vi "Regenerate Hawkeye List.vi"() -> ()   [LabVIEW 2019, in "HawkeyeToolsMenu.lvlib"]
doc: "GUI to compare LabVIEW code between currently checked out branch with any other branch or any of its commits.\n\n(c) 2024 Soliton Technologies. All rights reserved."
uses:
  <vilib>/Hampel Software Engineering/Git API/Git API/GIT-api.lvclass
  <vilib>/Hampel Software Engineering/Git API/Git API/GIT-api.lvclass/GIT-api.ctl
  <vilib>/Hampel Software Engineering/Git API/Git API/Controls/GIT-Repository States.ctl
  <vilib>/Hampel Software Engineering/Git API/Git API/Accessors/GIT-Set Working Dir.vi
  <userlib>/_OpenG.lib/file/file.llb/File Exists - Scalar__ogtk.vi
  <userlib>/_OpenG.lib/file/file.llb/Valid Path - Traditional__ogtk.vi
  HawkeyeToolsMenu.lvlib
  vi.lib/Hawkeye/Hawkeye.lvlib
panel:
  in  "Tab Control":T1(tab)=enum."Main UI"
  out "Current Status":string
  in  "LVLib / LVClass / Sub Folder Path":path
  out "Status Indicator":string
  in  "Check Changed Libraries Only?":bool
  in  "Branch to Compare":string(combo)
  in  "Refresh Current Branch":bool
  out "Current Branch":string="origin/main"
  out "Current Branch Status":string
  in  "Stop":bool
  in  "Repo / Workspace Folder Path":path
  in  "Generate":bool
  # "1. Checkout the branch of interest in your system using any method - Git command line, Desktop Git GUI Clients etc.,\n\n2. Specify the local Repository Path.\n\n3. Verify the current branch, its status and select a branch or commit based on the Compare Mode and click on Compare to display the file changes.\n\n4. Double click on a file to initiate LabVIEW code comparison.\n\n5. Once done with required comparisons, exit the tool by closing the window. The tool cleans up the temporary files added during comparison.\n\n\nNote:\n1. This tool uses LabVIEW's VI Comparison Tool which requires LabVIEW Professional Development System.\n2. It is recommended to not use other Git Clients actively when comparing files using this tool to avoid Git command related errors.\n3. It is recommended to commit all changes (working copy) before using this tool for comparison."
  # "This tool uses git diff command to identify the changes. Hence it is recommended to commit all the changes (working copy) to have them considered for comparison. For code comparison, this tool uses LabVIEW's built in VI Comparison Tool.\n\nExample: Identify changes in current branch when comparing with other branch\n\n---A---B---C---D    <== other branch\n               \\\n                 E---F      <== current branch\n\n1. We will need to identify only the file changes introduced by current branch. E and F commits are those changes in the above example (commits after the common ancestor B).\n2. For the identified file changes compare with the other branch (D) to see how it differs. These differences will be our current branch changelist.\n\nWhy only current branch changes?\nIt is most useful to see how the current branch will modify the files when it is getting merged. Best use case for displaying only current branch changelist will be for Pull Request reviews."
  # "1. Repository Path - Local repository path (the top level folder with '.git' hidden folder in it). Git API will be initialized for this repository.\n\n2. Current Branch - Currently checked out branch. The status of the current branch is also displayed at top right. Click Refresh button to update the current branch if it is changed in the system or received new changes via Git Pull.\n\n3. Compare Mode - Select the type of comparison. You can compare the current branch with another branch or with a particular commit of a selected branch.\n\nIn branch comparison mode, you can enter the branch name for comparison in Branch to Compare. Remote branches usually start with \"origin/\" and local branches do not have \"origin/\" prefix. The branch's recent commit is displayed in Recent Commit and its details in Commit Details for reference. \n\nIn commit comparison mode, the commits available in the branch selected in Select Branch are listed in Commit to Compare. For the commit selected in Commit to Compare, its details will be displayed in the Commit Details. Use Commits to Fetch to limit the number of commits obtained and improve the loading time.\n\n     Note: Git doesn't maintain information on when the branch is created. So, all the commits of the selected branch will be displayed (all the way up to the very first commit after repository creation). Without a limit, it increases loading time.\n\n4. Compare - Identifies the file changes and Current Branch Changelist table shows the list of all files that are different in the current branch compared to the branch/commit selected.\n\n     Note: The other branch/commit in comparison would have introduced its own changes that are not part of current branch. Those changes will not be displayed.\n\n5. Filter LabVIEW VI and Control Files - Filter files except VI and CTL files. These require LabVIEW to compare but project, library and classes are text files that can be easily reviewed in the desktop Git GUI clients or in Pull Request of Git web services.\n\n6. LabVIEW Compare Options - Options to decide what to compare in the code. Set the required options before initiating code compare.\n\n7. Double click on the file you wish to compare. LabVIEW opens the compare window for the file from the current branch and the file from the other branch/commit (file will be suffixed with TEMP). It may take a while if the VI/CTL have lot of dependencies to load. Having the project pre-opened and opening this tool from that instance may reduce the loading time. Note that the file from the other branch/commit in comparison may be missing its dependent files which may not be available in the current branch or deleted in the current branch commits. This will cause the file to be in a broken state but does not affect the comparison. Another reason for the broken state may be due to the parent library/class not recognizing this new file with the suffix but this as well will not affect the comparison.\n\n     Note: The files from other branch/commit are placed at the same location in the current branch so that the LabVIEW can load the dependencies appropriately.\n\n8. Viewed Status (mixed checkbox) - A tick mark appears for every file compared or opened. Use the mixed checkbox (below the Current Branch Changelist) to control status for all files.\n\n     Note: Viewed status is only a visual aid for tracking and does not have any other function other than that.\n\n9. Panel Close - Stops the tools execution after removing all the new files introduced into the current branch (TEMP files)."
  # "This GUI allows you to regenerate dependency lists for the entire repository or for a selected folder, LabVIEW library (.lvlib), or LabVIEW class (.lvclass), ensuring dependency information is up to date."
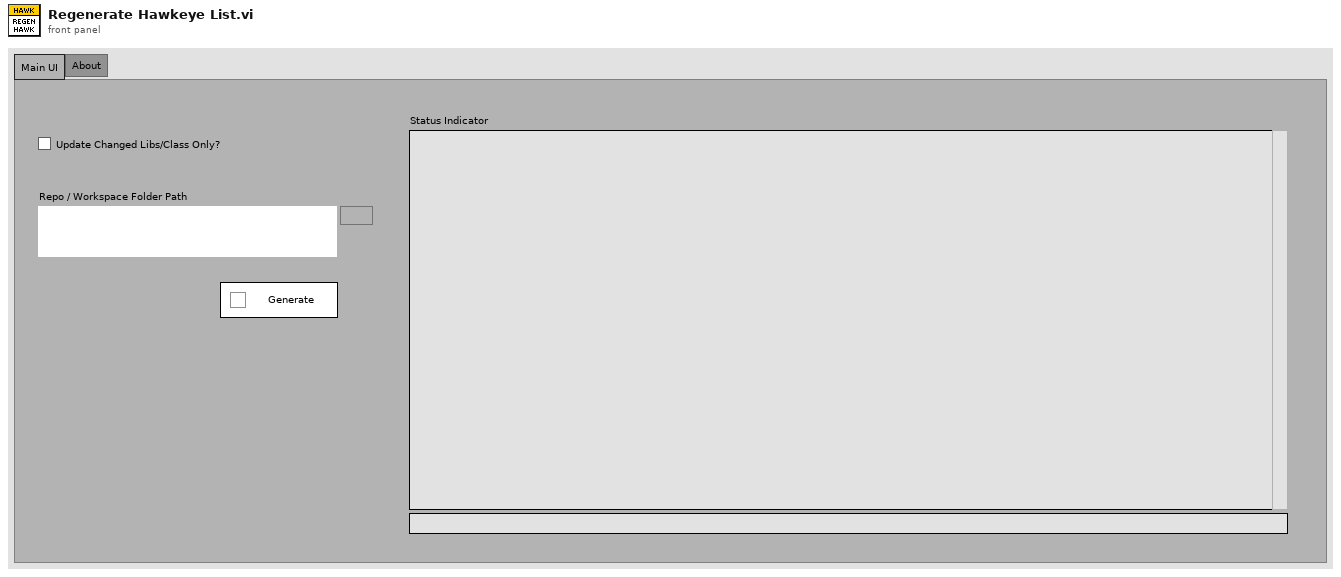
[diagram p1: front panel]
types:
  T1 = enum32{"Getting Started", "How it Works?", "Main UI", "Help", "About"}
  T2 = cluster{"Repository Path":path, "Git API Object":refnum<class "GIT-api.lvclass">, "Git API Initialized?":bool, "Current Branch":string, "Branch to Compare":string, "Check Changed Libraries Only?":bool, "Source Folder Path":path, "Build Specs Folder Path":path}
  T3 = typedef "GIT-API-for-LabVIEW.lvlib/GIT-api.lvclass/GIT-Repository States.ctl" = enum16{"up-to-date", "behind", "ahead", "diverged", "unpublished", "detached", "unknown"}
  T4 = enum8{"Enabled", "Disabled", "Disabled and Grayed Out"}
  T5 = typedef "Hawkeye.lvlib/HawkeyePathConfigs.ctl" = cluster{"GlobalIncludePaths":path[], "GlobalExcludePaths":path[], "BuildSpecsIncludePaths":path[], "ActualDepsIncludePaths":path[], "WorkspacePath":path, "SourceFolderPaths":path[], "ChangedFilesLogpaths":map{string, path}, "CacheRecreateDuration":dbl}
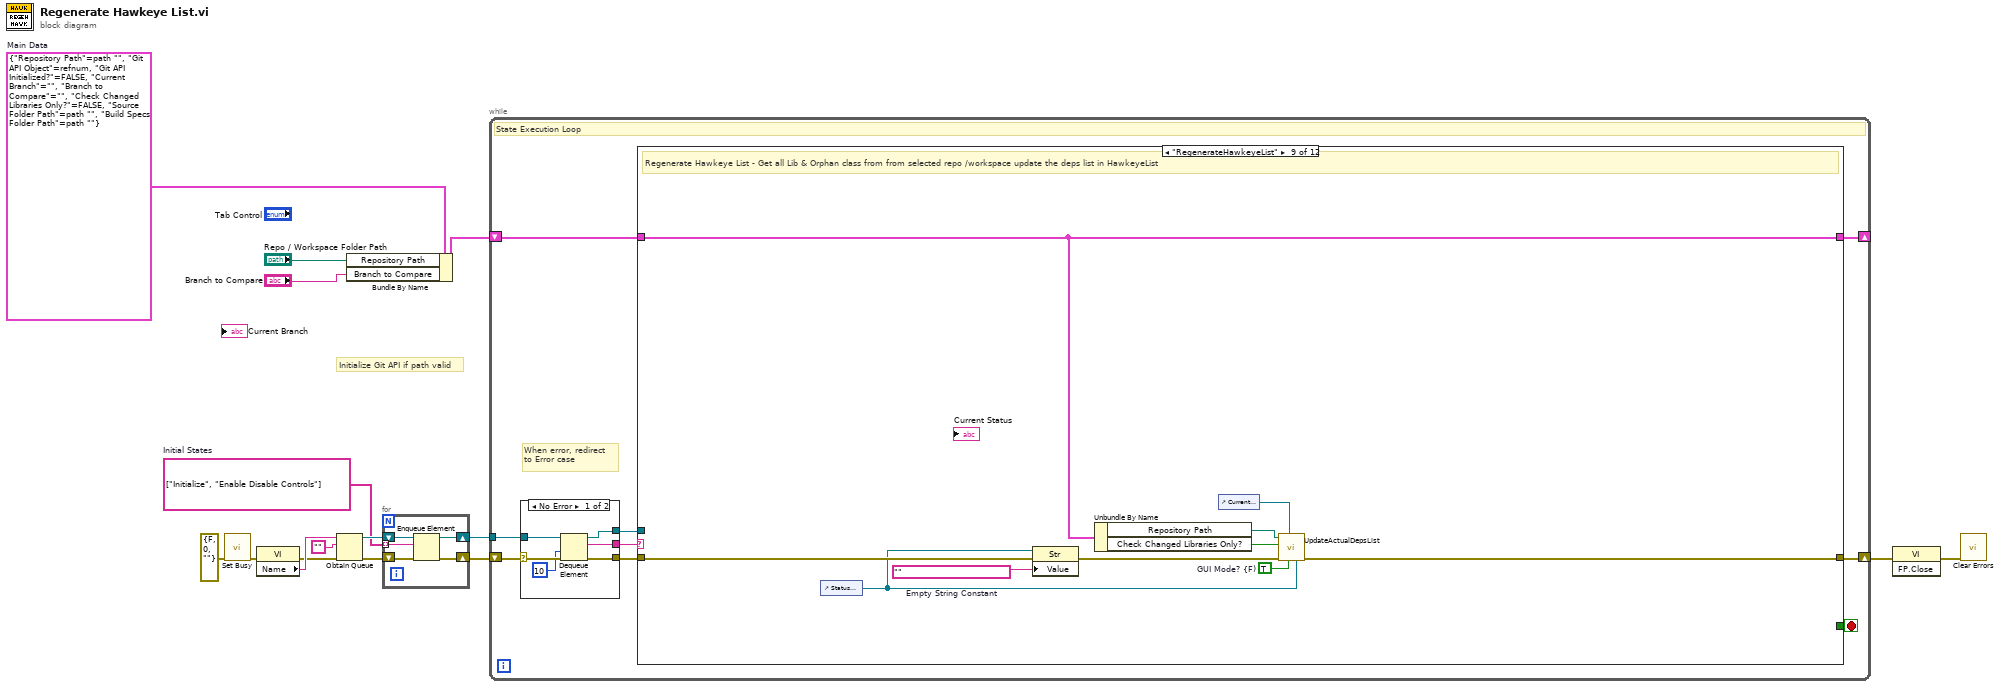
[diagram p0: block diagram]
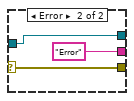
[diagram p2: hidden frame]
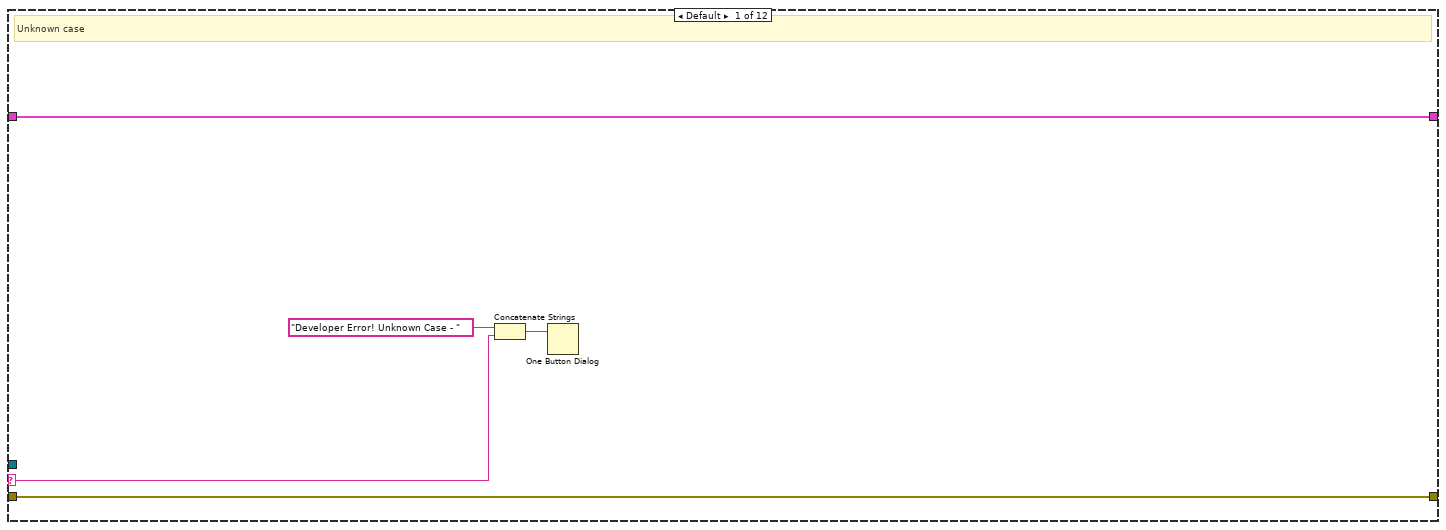
[diagram p3: hidden frame]
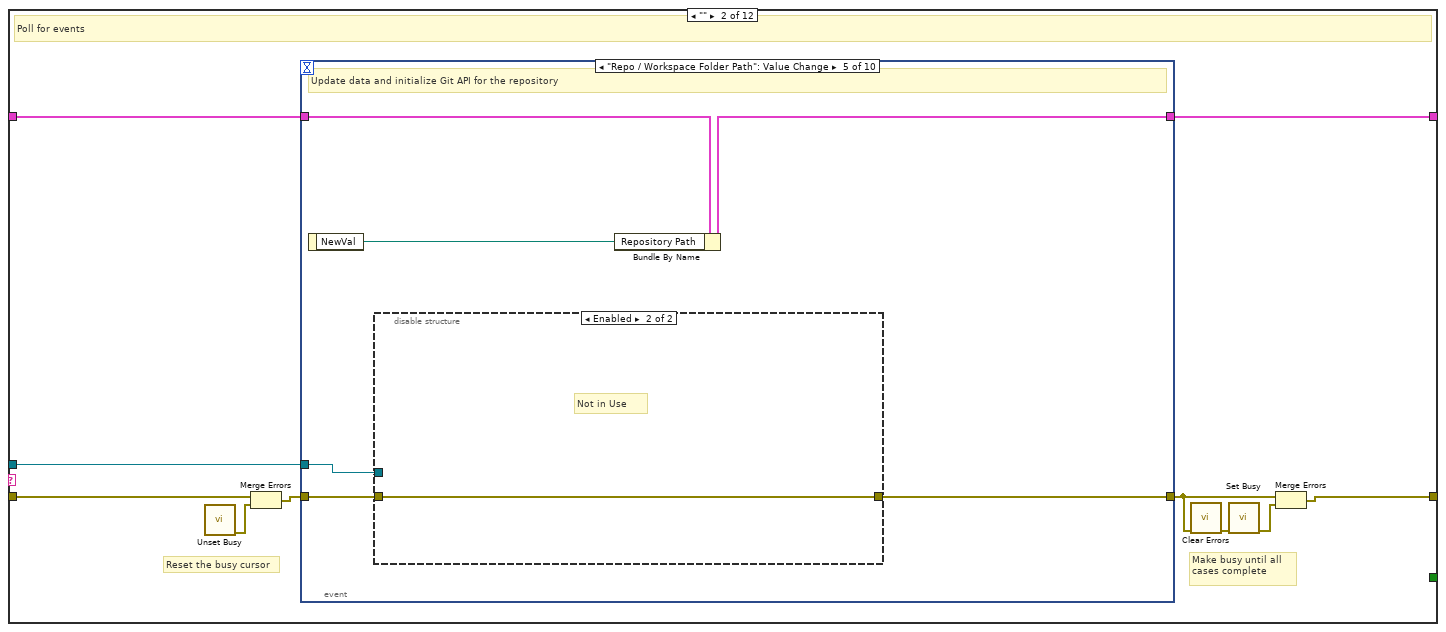
[diagram p4: hidden frame]
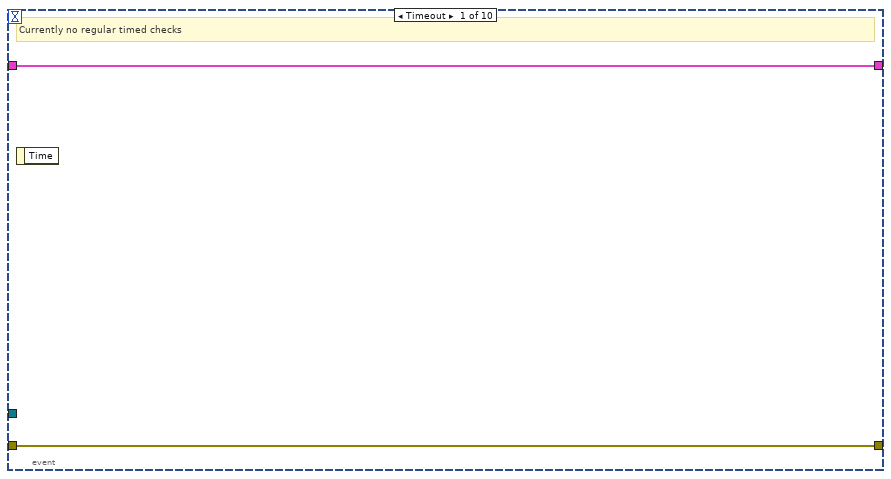
[diagram p5: hidden frame]
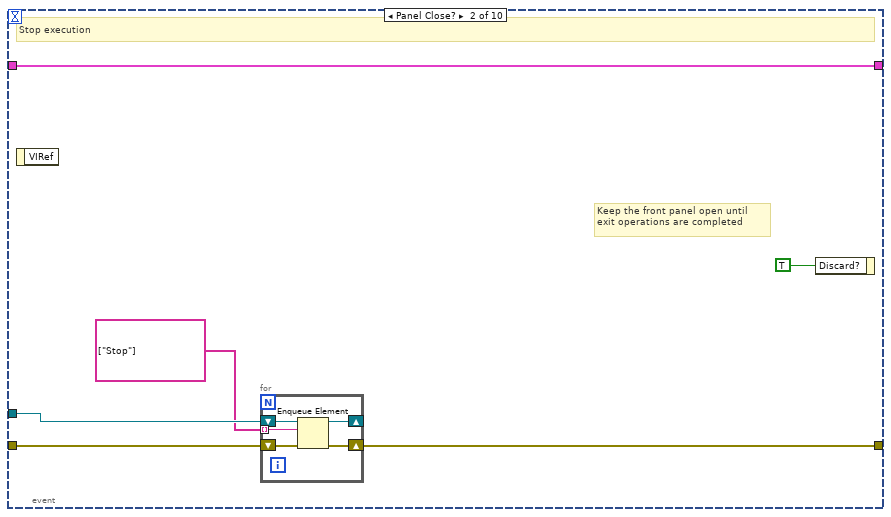
[diagram p6: hidden frame]
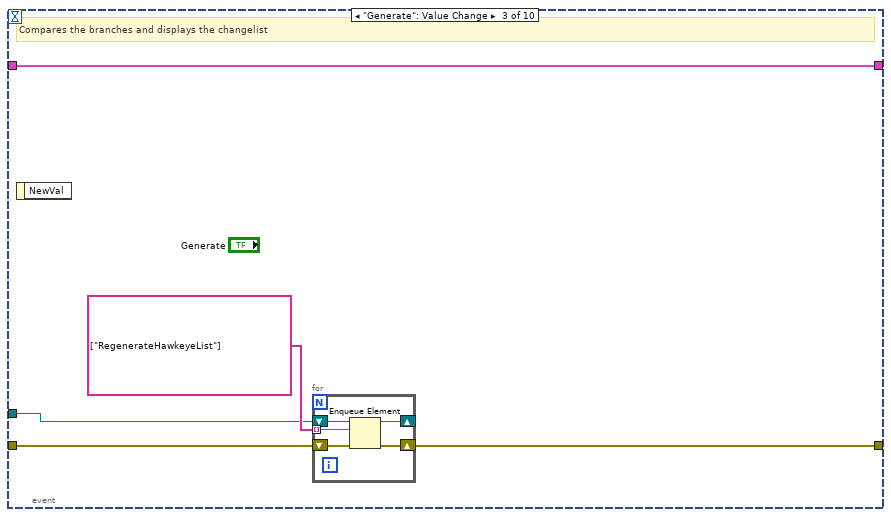
[diagram p7: hidden frame]
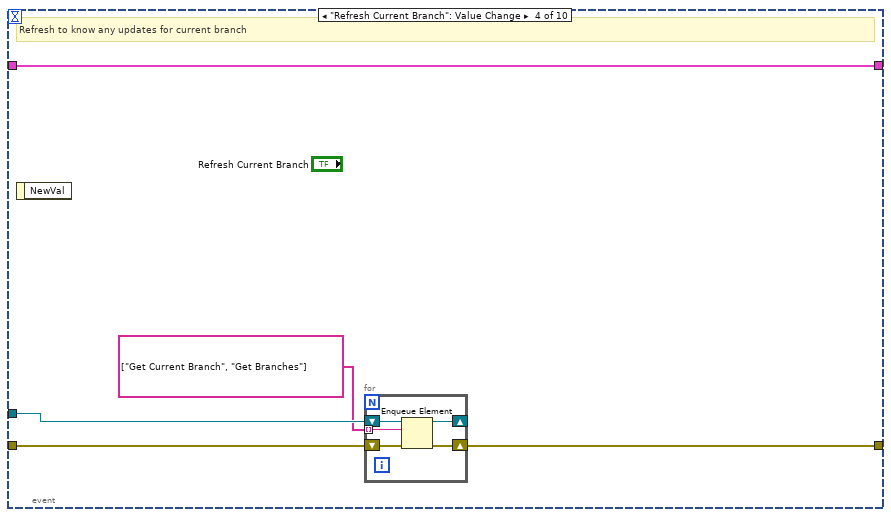
[diagram p8: hidden frame]
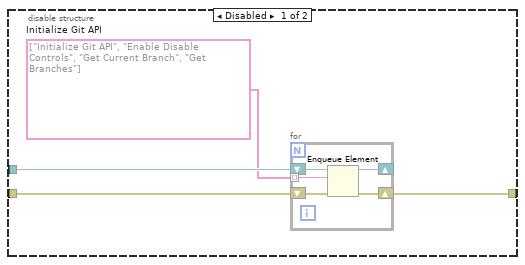
[diagram p9: hidden frame]
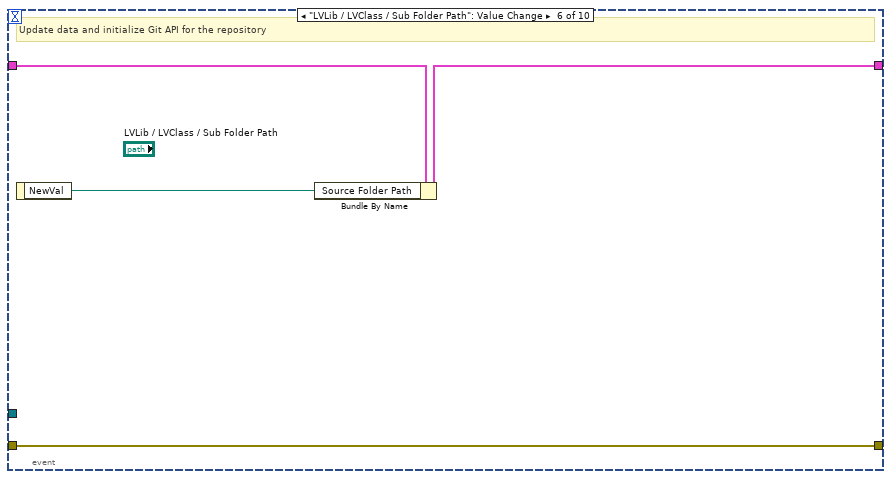
[diagram p10: hidden frame]
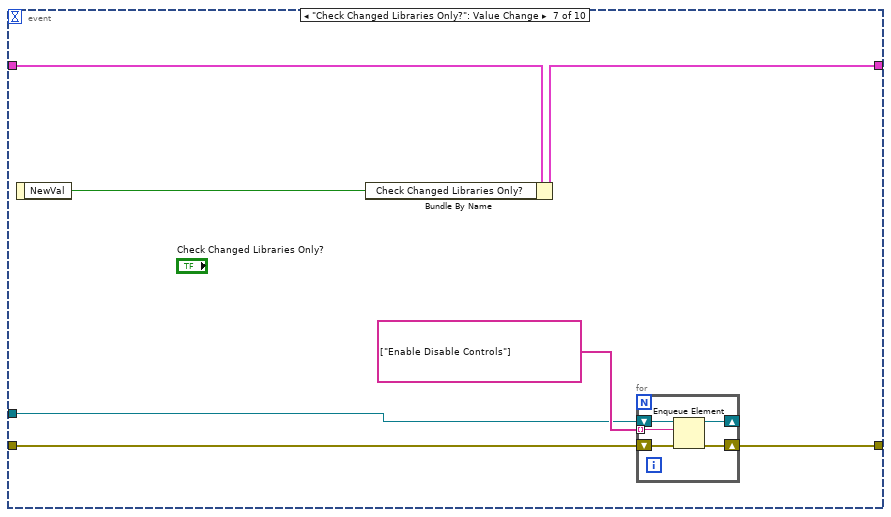
[diagram p11: hidden frame]
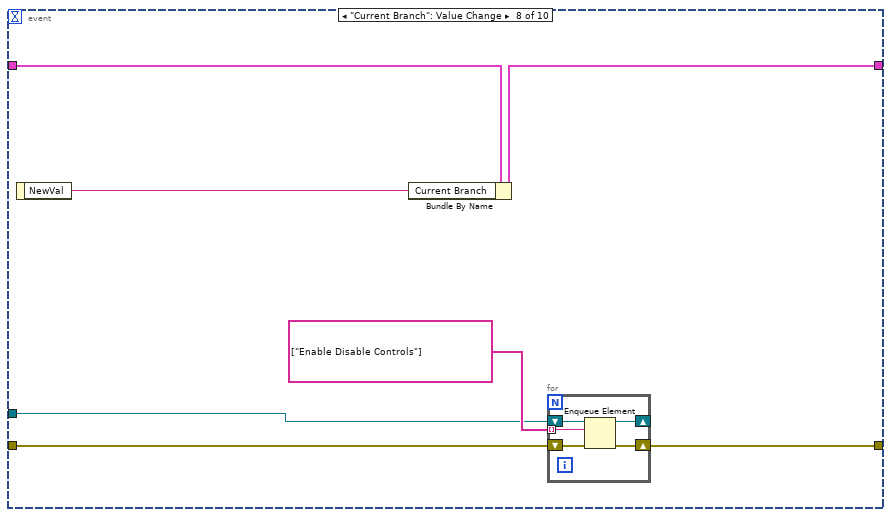
[diagram p12: hidden frame]
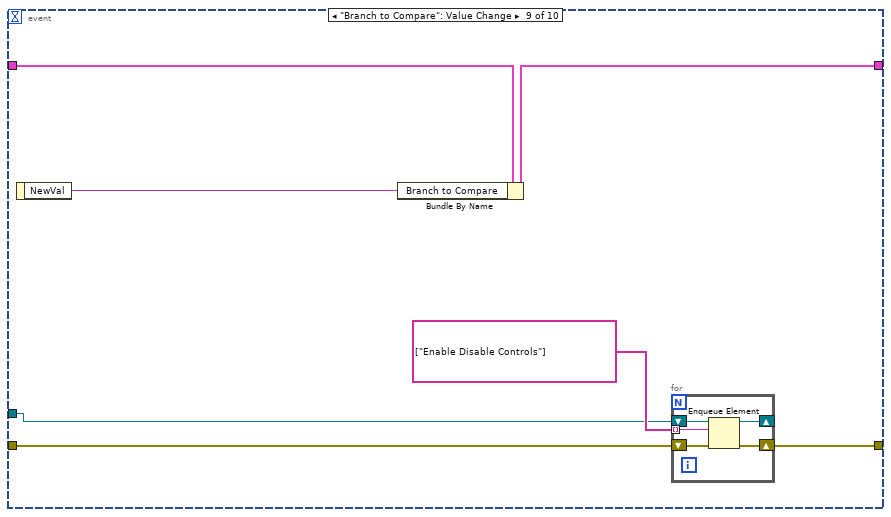
[diagram p13: hidden frame]
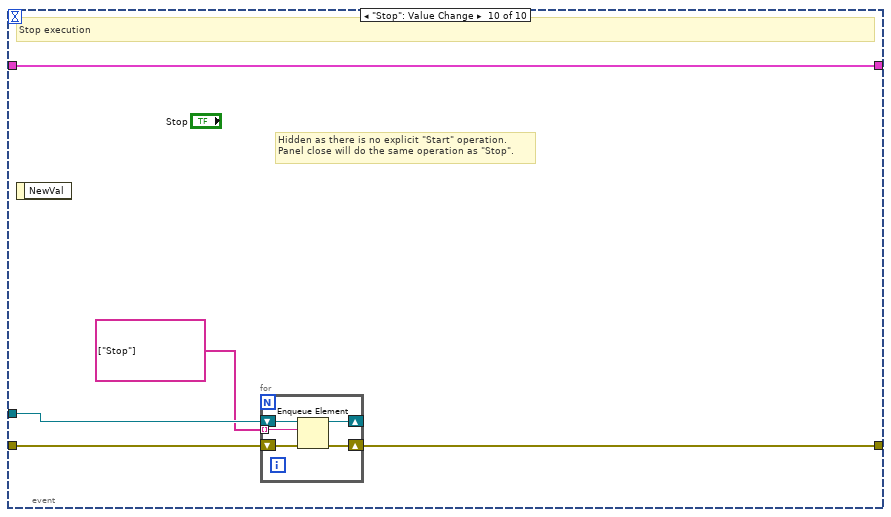
[diagram p14: hidden frame]
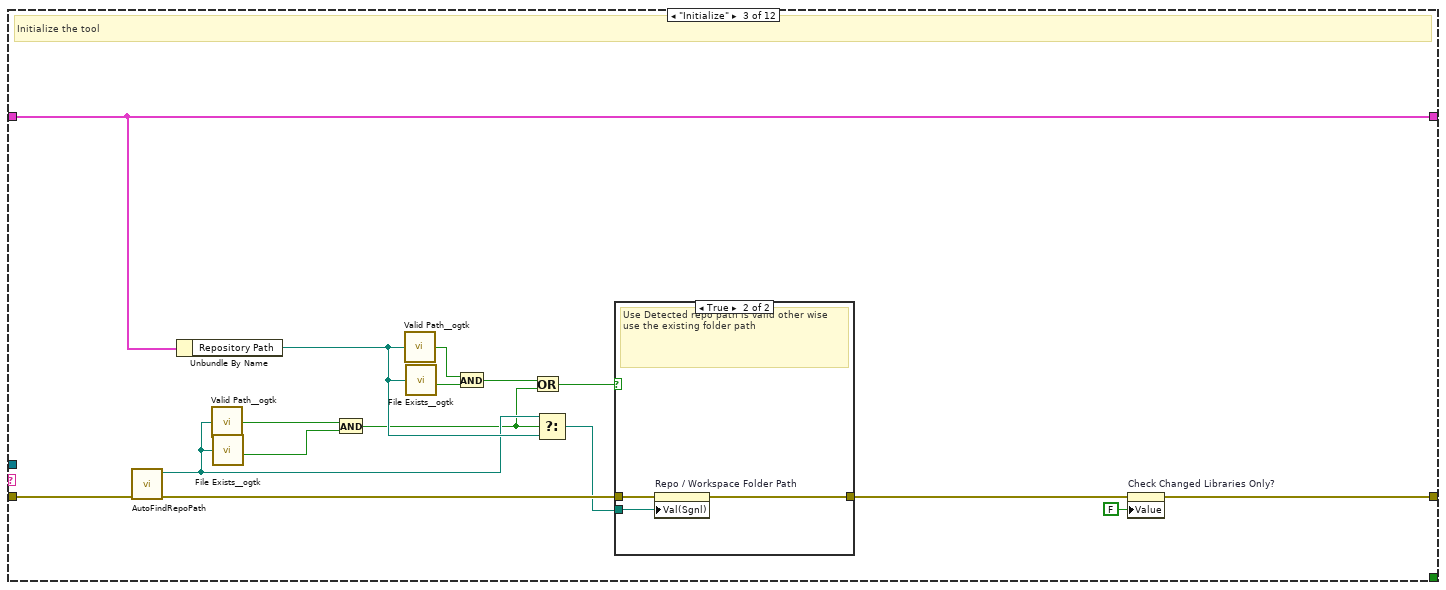
[diagram p15: hidden frame]
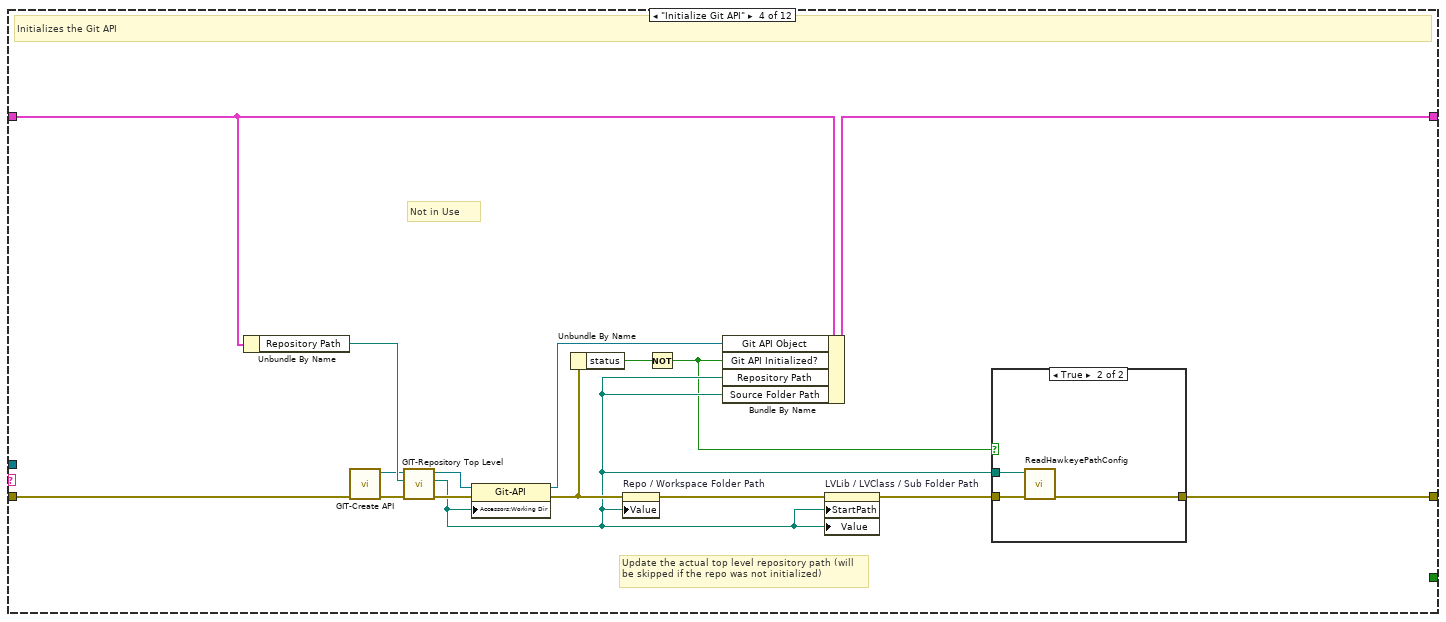
[diagram p17: hidden frame]
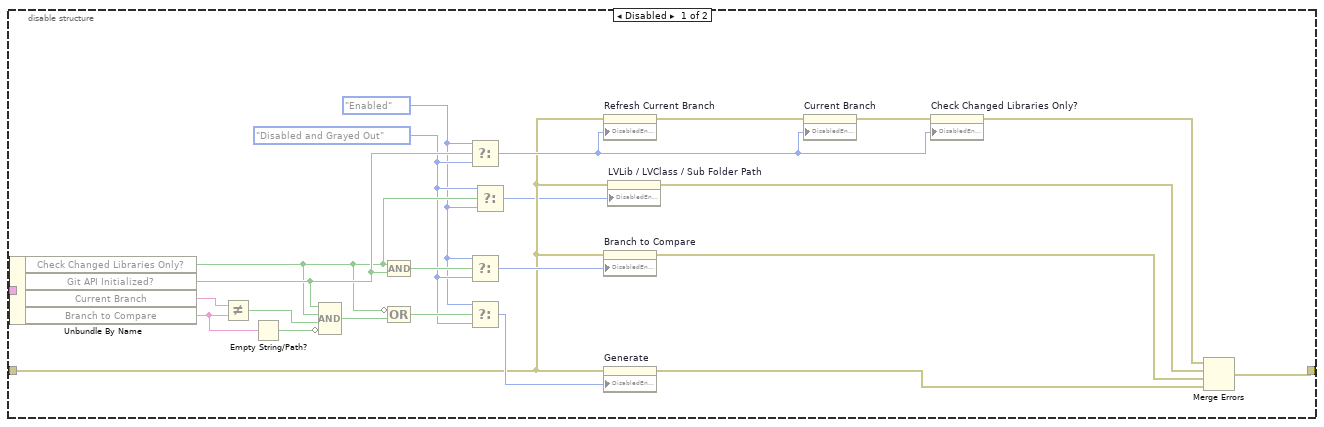
[diagram p20: hidden frame]
diagram:
  w1 = string[] ["Initialize", "Enable Disable Controls"]  # Initial States
  w13 = T2 {"Repository Path"=path "", "Git API Object"=refnum, "Git API Initialized?"=FALSE, "Current Branch"="", "Branch to Compare"="", "Check Changed Libraries Only?"=FALSE, "Source Folder Path"=path "", "Build Specs Folder Path"=path ""}  # Main Data
  # "Initialize Git API if path valid"
  n1 = call <vilib>:"Set Busy.vi"("error in (no error)"=errorcluster {"status"=FALSE, "code"=0, "source"=""}) -> ("error out"=w6:errorcluster)  [unwired: 9 in, 1 out]
  n2 = property class="VI"(error in=w6) -> (error out=w15:errorcluster, "Name"=w16:string)  [unwired: 1 in, 1 out]
  n3 = Obtain Queue(name (unnamed)=w16, element data type="", error in (no error)=w15) -> (queue out=w11:refnum<queue>, error out=w8:errorcluster)  [unwired: 2 in, 1 out]
  n4 = Bundle By Name(cluster=w13, "Repository Path"="Repo / Workspace Folder Path", "Branch to Compare"="Branch to Compare") -> (w12:T2)
  n5 = for {
    tunnel: w1 -> [w18] mode=indexing
    shift-right: [w20] -> w10
    shift-left: w8 -> [w21]
    shift-right: [w17] -> w9
    shift-left: w11 -> [w19]
    n6 = Enqueue Element(queue=w19, element=w18, error in (no error)=w21) -> (queue out=w17:refnum<queue>, error out=w20:errorcluster)  [unwired: 1 in, 1 out]
  }
  n7 = while {
    shift-right: [w22] -> w4
    shift-left: w10 -> [w24]
    tunnel: w9 -> [w25]
    shift-right: [w27] -> _
    shift-left: w12 -> [w26]
    stop <- w28 stop-if-true
    # "When error, redirect to Error case"
    # "State Execution Loop"
    n8 = case shown="No Error" w24 {
      selector: w24 -> [w33 w37]
      tunnel: [w36 "Error" ("element")] -> w30
      tunnel: [w35 w39] -> w29
      tunnel: w25 -> [w34 w39]
      tunnel: [w31 w37] -> w23
      frame No Error {
        n9 = Dequeue Element(queue=w34, timeout in ms (-1)=10, error in (no error)=w33) -> (queue out=w35:refnum<queue>, element=w36:string, error out=w31:errorcluster)  [unwired: 1 out]
      }
      frame Error {
      }
    }
    n10 = case shown="\"RegenerateHawkeyeList\"" w30 {
      selector: w30 -> [w43 _ _ _ _ _ _ _ _ _ _ _]
      tunnel: w23 -> [w41 w48 w166 w189 w194 w227 w273 w303 w324 w333 w343 w351]
      tunnel: w29 -> [_ w54 _ _ _ _ _ _ _ w331 w340 w348]
      tunnel: [w41 w50 w169 w175 w195 w236 w282 w299 w325 w332 w339 w344] -> w22
      tunnel: [_ _ _ _ _ _ _ _ _ _ w341 _] -> w28
      tunnel: [w40 w52 w163 w186 w196 w239 w280 w304 w328 w330 w342 w352] -> w27
      tunnel: w26 -> [w40 w53 w163 w188 w196 w240 w281 w304 w328 w330 w342 w352]
      frame Default {
        # "Unknown case"
        n11 = Concatenate Strings("Developer Error! Unknown Case - " ("string"), w43) -> (w42:string)
        n12 = One Button Dialog(message=w42) -> ()  [unwired: 1 in, 1 out]
      }
      frame "" {
        # "Reset the busy cursor"
        # "Make busy until all cases complete"
        # "Poll for events"
        n13 = call <vilib>:"Unset Busy.vi"() -> ("error out"=w49:errorcluster)  [unwired: 11 in]
        n14 = Merge Errors(w48, w49) -> (w47:errorcluster)
        n15 = event shown="[4] \"Repo / Workspace Folder Path\": Value Change" {
          selector: _ -> [_ _ _ _ _ _ _ _ _ _]
          dyn-events: _ -> [_ _ _ _ _ _ _ _ _ _]
          timeout: _ -> [_ _ _ _ _ _ _ _ _ _]
          tunnel: w47 -> [w55 w62 w71 w82 w90 w104 w109 w120 w132 w148]
          tunnel: w54 -> [_ w61 w70 w81 w89 _ w108 w122 w134 w147]
          tunnel: [w55 w60 w69 w79 w88 w104 w110 w121 w133 w146] -> w46
          tunnel: w53 -> [w56 w59 w68 w78 w93 w107 w114 w126 w138 w145]
          tunnel: [w56 w59 w68 w78 w92 w106 w113 w125 w137 w145] -> w52
          event Timeout {
            # "Currently no regular timed checks"
            n16 = event-data() -> ()  [unwired: 1 in, 1 out]
          }
          event Panel Close? {
            # "Keep the front panel open until exit operations are completed"
            # "Stop execution"
            n17 = event-data() -> ()  [unwired: 1 in, 1 out]
            n18 = for {
              tunnel: string[] ["Stop"] -> [w64] mode=indexing
              shift-right: [w66] -> w60
              shift-left: w62 -> [w67]
              shift-right: [w63] -> _
              shift-left: w61 -> [w65]
              n19 = Enqueue Element(queue=w65, element=w64, error in (no error)=w67) -> (queue out=w63:refnum<queue>, error out=w66:errorcluster)  [unwired: 1 in, 1 out]
            }
            n20 = event-data("Discard?"=TRUE) -> ()  [unwired: 1 in, 1 out]
          }
          event "Generate": Value Change {
            # "Compares the branches and displays the changelist"
            n21 = event-data() -> ()  [unwired: 1 in, 1 out]
            n22 = for {
              tunnel: string[] ["RegenerateHawkeyeList"] -> [w74] mode=indexing
              shift-right: [w76] -> w69
              shift-left: w71 -> [w77]
              shift-right: [w73] -> _
              shift-left: w70 -> [w75]
              n23 = Enqueue Element(queue=w75, element=w74, error in (no error)=w77) -> (queue out=w73:refnum<queue>, error out=w76:errorcluster)  [unwired: 1 in, 1 out]
            }
          }
          event "Refresh Current Branch": Value Change {
            # "Refresh to know any updates for current branch"
            n24 = event-data() -> ()  [unwired: 1 in, 1 out]
            n25 = for {
              tunnel: string[] ["Get Current Branch", "Get Branches"] -> [w84] mode=indexing
              shift-right: [w86] -> w79
              shift-left: w82 -> [w87]
              shift-right: [w83] -> _
              shift-left: w81 -> [w85]
              n26 = Enqueue Element(queue=w85, element=w84, error in (no error)=w87) -> (queue out=w83:refnum<queue>, error out=w86:errorcluster)  [unwired: 1 in, 1 out]
            }
          }
          event "Repo / Workspace Folder Path": Value Change {
            # "Update data and initialize Git API for the repository"
            n27 = event-data() -> ("NewVal"=w91:path)  [unwired: 1 in]
            n28 = disable-structure shown="Enabled" {
              disable-tunnel: w90 -> [w97 w103]
              disable-tunnel: w89 -> [w96 _]
              disable-tunnel: [w95 w103] -> w88
              frame Disabled {
                w94 = string[] ["Initialize Git API", "Enable Disable Controls", "Get Current Branch", "Get Branches"]  # Initialize Git API
                n29 = for {
                  tunnel: w94 -> [w99] mode=indexing
                  shift-right: [w101] -> w95
                  shift-left: w97 -> [w102]
                  shift-right: [w98] -> _
                  shift-left: w96 -> [w100]
                  n30 = Enqueue Element(queue=w100, element=w99, error in (no error)=w102) -> (queue out=w98:refnum<queue>, error out=w101:errorcluster)  [unwired: 1 in, 1 out]
                }
              }
              frame Enabled {
                # "Not in Use"
              }
            }
            n31 = Bundle By Name(cluster=w93, "Repository Path"=w91) -> (w92:T2)
          }
          event "LVLib / LVClass / Sub Folder Path": Value Change {
            # "Update data and initialize Git API for the repository"
            n32 = event-data() -> ("NewVal"=w105:path)  [unwired: 1 in]
            n33 = Bundle By Name(cluster=w107, "Source Folder Path"=w105) -> (w106:T2)
          }
          event "Check Changed Libraries Only?": Value Change {
            n34 = event-data() -> ("NewVal"=w112:bool)  [unwired: 1 in]
            n35 = Bundle By Name(cluster=w114, "Check Changed Libraries Only?"=w112) -> (w113:T2)
            n36 = for {
              tunnel: string[] ["Enable Disable Controls"] -> [w116] mode=indexing
              shift-right: [w118] -> w110
              shift-left: w109 -> [w119]
              shift-right: [w115] -> _
              shift-left: w108 -> [w117]
              n37 = Enqueue Element(queue=w117, element=w116, error in (no error)=w119) -> (queue out=w115:refnum<queue>, error out=w118:errorcluster)  [unwired: 1 in, 1 out]
            }
          }
          event "Current Branch": Value Change {
            n38 = event-data() -> ("NewVal"=w124:string)  [unwired: 1 in]
            n39 = Bundle By Name(cluster=w126, "Current Branch"=w124) -> (w125:T2)
            n40 = for {
              tunnel: string[] ["Enable Disable Controls"] -> [w128] mode=indexing
              shift-right: [w130] -> w121
              shift-left: w120 -> [w131]
              shift-right: [w127] -> _
              shift-left: w122 -> [w129]
              n41 = Enqueue Element(queue=w129, element=w128, error in (no error)=w131) -> (queue out=w127:refnum<queue>, error out=w130:errorcluster)  [unwired: 1 in, 1 out]
            }
          }
          event "Branch to Compare": Value Change {
            n42 = event-data() -> ("NewVal"=w136:string)  [unwired: 1 in]
            n43 = Bundle By Name(cluster=w138, "Branch to Compare"=w136) -> (w137:T2)
            n44 = for {
              tunnel: string[] ["Enable Disable Controls"] -> [w140] mode=indexing
              shift-right: [w142] -> w133
              shift-left: w132 -> [w143]
              shift-right: [w139] -> _
              shift-left: w134 -> [w141]
              n45 = Enqueue Element(queue=w141, element=w140, error in (no error)=w143) -> (queue out=w139:refnum<queue>, error out=w142:errorcluster)  [unwired: 1 in, 1 out]
            }
          }
          event "Stop": Value Change {
            # "Hidden as there is no explicit \"Start\" operation.\nPanel close will do the same operation as \"Stop\"."
            # "Stop execution"
            n46 = event-data() -> ()  [unwired: 1 in, 1 out]
            n47 = for {
              tunnel: string[] ["Stop"] -> [w150] mode=indexing
              shift-right: [w152] -> w146
              shift-left: w148 -> [w153]
              shift-right: [w149] -> _
              shift-left: w147 -> [w151]
              n48 = Enqueue Element(queue=w151, element=w150, error in (no error)=w153) -> (queue out=w149:refnum<queue>, error out=w152:errorcluster)  [unwired: 1 in, 1 out]
            }
          }
        }
        n49 = call <vilib>:"Clear Errors.vi"("error in (no error)"=w46) -> ("error out"=w45:errorcluster)  [unwired: 5 in, 1 out]
        n50 = call <vilib>:"Set Busy.vi"("error in (no error)"=w45) -> ("error out"=w51:errorcluster)  [unwired: 9 in, 1 out]
        n51 = Merge Errors(w46, w51) -> (w50:errorcluster)
      }
      frame "Initialize" {
        # "Initialize the tool"
        n52 = call "AutoFindRepoPath.vi"("error in (no error)"=w166) -> ("error out"=w167:errorcluster, "Repo Path"=w157:path)  [unwired: 9 in]
        n53 = Unbundle By Name(w163) -> ("Repository Path"=w159:path)
        n54 = call-poly <userlib>:"Valid Path__ogtk.vi"("path"=w157) -> ("valid"=w164:bool)
        n55 = call-poly <userlib>:"File Exists__ogtk.vi"("file path"=w157) -> ("exists"=w165:bool)  [unwired: 6 in, 1 out]
        n56 = And(x=w164, y=w165) -> (x .and. y?=w156:bool)
        n57 = call-poly <userlib>:"Valid Path__ogtk.vi"("path"=w159) -> ("valid"=w158:bool)
        n58 = call-poly <userlib>:"File Exists__ogtk.vi"("file path"=w159) -> ("exists"=w162:bool)  [unwired: 6 in, 1 out]
        n59 = And(x=w158, y=w162) -> (x .and. y?=w161:bool)
        n60 = Or(x=w161, y=w156) -> (x .or. y?=w160:bool)
        n61 = Select(t=w157, s=w156, f=w159) -> (s? t:f=w154:path)
        n62 = case shown="True" w160 {
          tunnel: w167 -> [w170 w173]
          tunnel: [w170 w171] -> w155
          tunnel: w154 -> [_ w172]
          frame False {
          }
          frame True {
            # "Use Detected repo path is valid other wise use the existing folder path"
            n63 = property on="Repo / Workspace Folder Path" class="Path"(error in=w173, "Val(Sgnl)"=w172) -> (error out=w171:errorcluster)  [unwired: 1 in, 1 out]
          }
        }
        n64 = property on="Check Changed Libraries Only?" class="Bool (strict)"(error in=w155, "Value"=FALSE ("Check Changed Libraries Only?")) -> (error out=w169:errorcluster)  [unwired: 1 in, 1 out]
      }
      frame "Initialize Git API" {
        # "Not in Use"
        # "Update the actual top level repository path (will be skipped if the repo was not initialized)"
        # "Initializes the Git API"
        n65 = Unbundle By Name(w188) -> ("Repository Path"=w185:path)
        n66 = call <vilib>:"GIT-Create API.vi"("error in"=w189) -> ("error out"=w184:errorcluster, "git-api out"=w182:refnum<class "GIT-api.lvclass">)  [unwired: 9 in]
        n67 = call <vilib>:"GIT-Repository Top Level.vi"("error in"=w184, "Current Path"=w185, "git-api in"=w182) -> ("error out"=w181:errorcluster, "Repo Top Level Path"=w177:path, "git-api out"=w183:refnum<class "GIT-api.lvclass">)  [unwired: 6 in]
        n68 = property class="Git-API"(reference=w183, error in=w181, "Accessors:Working Dir"=w177) -> (reference out=w187:refnum<class "GIT-api.lvclass">, error out=w179:errorcluster)
        n69 = Unbundle By Name(w179) -> ("status"=w180:bool)
        n70 = property on="Repo / Workspace Folder Path" class="Path"(error in=w179, "Value"=w177) -> (error out=w178:errorcluster)  [unwired: 1 in, 1 out]
        n71 = Not(x=w180) -> (.not. x?=w174:bool)
        n72 = Bundle By Name(cluster=w188, "Git API Object"=w187, "Git API Initialized?"=w174, "Repository Path"=w177, "Source Folder Path"=w177) -> (w186:T2)
        n73 = property on="LVLib / LVClass / Sub Folder Path" class="Path"(error in=w178, "StartPath"=w177, "Value"=w177) -> (error out=w176:errorcluster)  [unwired: 1 in, 1 out]
        n74 = case shown="True" w174 {
          tunnel: w177 -> [_ w193]
          tunnel: w176 -> [w190 w192]
          tunnel: [w190 w191] -> w175
          frame False {
          }
          frame True {
            n75 = call "ReadHawkeyePathConfig.vi"("error in (no error)"=w192, "Workspace Path"=w193) -> ("error out"=w191:errorcluster)  [unwired: 8 in, 1 out]
          }
        }
      }
      frame "Enable Disable Controls" {
        # "Enable or disable controls based on Git API initialized or not"
        n76 = disable-structure shown="Enabled" {
          disable-tunnel: w196 -> [w220 _]
          disable-tunnel: [w219 w221] -> w195
          disable-tunnel: w194 -> [w202 w221]
          frame Disabled {
            w199 = T4."Disabled and Grayed Out" ("Disabled")
            w198 = T4."Enabled" ("Disabled")
            n77 = Unbundle By Name(w220) -> ("Check Changed Libraries Only?"=w200:bool, "Git API Initialized?"=w207:bool, "Current Branch"=w215:string, "Branch to Compare"=w211:string)
            n78 = Not Equal?(x=w215, y=w211) -> (x != y?=w208:bool)
            n79 = Empty String/Path?(string/path=w211) -> (empty?=w210:bool)
            n80 = Compound Arithmetic op=AND(w207, w200, w208, invert w210) -> (w209:bool)
            n81 = Compound Arithmetic op=AND(w200, w207) -> (w214:bool)
            n82 = Compound Arithmetic op=OR(invert w200, w209) -> (w216:bool)
            n83 = Select(t=w198, s=w207, f=w199) -> (s? t:f=w203:T4)
            n84 = Select(t=w198, s=w214, f=w199) -> (s? t:f=w213:T4)
            n85 = Select(t=w198, s=w216, f=w199) -> (s? t:f=w217:T4)
            n86 = Select(t=w199, s=w200, f=w198) -> (s? t:f=w197:T4)
            n87 = property on="Refresh Current Branch" class="Bool"(error in=w202, "DisabledEnum"=w203) -> (error out=w206:errorcluster)  [unwired: 1 in, 1 out]
            n88 = property on="Branch to Compare" class="CmbBox"(error in=w202, "DisabledEnum"=w213) -> (error out=w218:errorcluster)  [unwired: 1 in, 1 out]
            n89 = property on="Generate" class="Bool"(error in=w202, "DisabledEnum"=w217) -> (error out=w212:errorcluster)  [unwired: 1 in, 1 out]
            n90 = property on="LVLib / LVClass / Sub Folder Path" class="Path"(error in=w202, "DisabledEnum"=w197) -> (error out=w201:errorcluster)  [unwired: 1 in, 1 out]
            n91 = property on="Current Branch" class="Str"(error in=w206, "DisabledEnum"=w203) -> (error out=w205:errorcluster)  [unwired: 1 in, 1 out]
            n92 = property on="Check Changed Libraries Only?" class="Bool (strict)"(error in=w205, "DisabledEnum"=w203) -> (error out=w204:errorcluster)  [unwired: 1 in, 1 out]
            n93 = Merge Errors(w204, w201, w218, w212) -> (w219:errorcluster)
          }
          frame Enabled {
            # "Not in Use"
          }
        }
      }
      frame "Get Current Branch" {
        # "Not in Use"
        # "Fetch updates from all remotes"
        # "Identify the currently checked out branch and its status and update the UI control"
        n94 = Unbundle By Name(w240) -> ("Git API Object"=w228:refnum<class "GIT-api.lvclass">)
        n95 = call <vilib>:"GIT-Fetch.vi"("param"="--all", "error in"=w227, "git-api in"=w228) -> ("error out"=w233:errorcluster, "git-api out"=w234:refnum<class "GIT-api.lvclass">)  [unwired: 6 in, 1 out]
        n96 = call <vilib>:"GIT-Repository Status.vi"("error in"=w233, "git-api in"=w234) -> ("error out"=w242:errorcluster, "State"=w225:T3, "git-api out"=w241:refnum<class "GIT-api.lvclass">)  [unwired: 6 in, 1 out]
        n97 = call <vilib>:"GIT-Current Branch.vi"("error in"=w242, "git-api in"=w241) -> ("error out"=w226:errorcluster, "current branch"=w229:string)  [unwired: 7 in, 1 out]
        n98 = Equal?(x=GIT-Repository_States."detached", y=w225) -> (x = y?=w230:bool)
        n99 = Select(t="HEAD", s=w230, f=w229) -> (s? t:f=w222:string)
        n100 = Format Into String(format string="%s", error in=w226, w225) -> (resulting string=→"Current Branch Status":string, error out=w223:errorcluster)  [unwired: 1 in]
        n101 = case "Color for quick identification" shown="\"up-to-date\"" w225 {
          tunnel: [u32 32768 u32 16711680 u32 16860 u32 16744448 u32 16777222 u32 7171459 u32 16711680] -> w235
          frame "up-to-date" {
          }
          frame "behind" {
          }
          frame "ahead" {
          }
          frame "diverged" {
          }
          frame "unpublished" {
          }
          frame "detached" {
          }
          frame "unknown" {
          }
        }
        n102 = Bundle By Name(cluster=w240, "Current Branch"=w222) -> (w239:T2)
        n103 = property on="Current Branch Status" class="Str"(error in=w223, "Text.TextColor"=w235) -> (error out=w236:errorcluster)  [unwired: 1 in, 1 out]
      }
      frame "Get Branches" {
        w263 = 0  # Branch Name List
        w268 = string[][] []
        w267 = "%s" ("format string")
        # "Not in Use"
        # "Reset if previous value not found"
        # "Combine local and remote branches"
        # "List Local branches"
        # "List Remote branches\nNote: All remote branches usually start with origin/ unless renamed"
        # "Reset if previous value not found"
        # "Get all local and remote branches and update UI control"
        n104 = Unbundle By Name(w281) -> ("Current Branch"=w253:string, "Git API Object"=w271:refnum<class "GIT-api.lvclass">)
        n105 = call <vilib>:"GIT-Branch.vi"("error in"=w273, "git-api in"=w271) -> ("error out"=w272:errorcluster, "std out"=w264:string, "git-api out"=w265:refnum<class "GIT-api.lvclass">)  [unwired: 7 in]
        n106 = call <vilib>:"GIT-Branch.vi"("param"="-r", "error in"=w272, "git-api in"=w265) -> ("error out"=w275:errorcluster, "std out"=w266:string)  [unwired: 6 in, 1 out]
        n107 = Spreadsheet String To Array(format string=w267, spreadsheet string=w264, array type (2D Dbl)=w268) -> (array=w283:string[][])  [unwired: 1 in]
        n108 = Spreadsheet String To Array(format string=w267, spreadsheet string=w266, array type (2D Dbl)=w268) -> (array=w269:string[][])  [unwired: 1 in]
        n109 = Index Array(array=w283, index (col)=w263) -> (element=w270:string[])  [unwired: 1 in]
        n110 = Index Array(array=w269, index (col)=w263) -> (element=w259:string[])  [unwired: 1 in]
        n111 = for "Remove current branch pointer" {
          tunnel: w270 -> [w292] mode=indexing
          tunnel: [w288] -> w262 mode=indexing
          tunnel: [w287] -> w284 mode=indexing
          n112 = Search and Replace String(input string=w292, search string="*", replace string="") -> (result string=w289:string, error out=w287:errorcluster)  [unwired: 5 in, 2 out]
          n113 = call <vilib>:"Trim Whitespace.vi"("string"=w289) -> ("trimmed string"=w288:string)  [unwired: 1 in]
        }
        n114 = for {
          tunnel: [w286] -> w260 mode=indexing
          tunnel: w259 -> [w285] mode=indexing
          n115 = call <vilib>:"Trim Whitespace.vi"("string"=w285) -> ("trimmed string"=w286:string)  [unwired: 1 in]
        }
        n116 = Build Array (concatenate)(w262, w260) -> (w254:string[])
        n117 = Merge Errors(w275, w284) -> (w261:errorcluster)
        n118 = Search 1D Array(1D array=w254, element=w253) -> (index of element=w256:i32)  [unwired: 1 in]
        n119 = Greater Or Equal To 0?(x=w256) -> (x >= 0?=w257:bool)
        n120 = Select(t=w253, s=w257, f="") -> (s? t:f=w255:string)
        n121 = property on="Current Branch" class="Str"(error in=w261, "Value"=w255) -> (error out=w252:errorcluster)  [unwired: 1 in, 1 out]
        n122 = property on="Branch to Compare" class="CmbBox"(error in=w252, "Strings[]"=w254) -> (error out=w251:errorcluster, "Value"=w250:string)  [unwired: 1 in, 1 out]
        n123 = Search 1D Array(1D array=w254, element=w250) -> (index of element=w279:i32)  [unwired: 1 in]
        n124 = Greater Or Equal To 0?(x=w279) -> (x >= 0?=w278:bool)
        n125 = Select(t=w250, s=w278, f="") -> (s? t:f=w276:string)
        n126 = Bundle By Name(cluster=w281, "Branch to Compare"=w276) -> (w280:T2)
        n127 = property on="Branch to Compare" class="CmbBox"(error in=w251, "Value"=w276) -> (error out=w282:errorcluster)  [unwired: 1 in, 1 out]
      }
      frame "RegenerateHawkeye" {
        w305 = TRUE  # GUI Mode? {F)
        # "Not in Use"
        # "Update the list is exist files"
        n128 = Unbundle By Name(w304) -> ("Repository Path"=w296:path, "Source Folder Path"=w297:path, "Check Changed Libraries Only?"=w298:bool, "Current Branch"=w302:string, "Branch to Compare"=w301:string)
        n129 = case shown="True" w298 {
          tunnel: [w306 w317] -> w300
          tunnel: w305 -> [_ w316]
          tunnel: w296 -> [_ w311]
          tunnel: w303 -> [w306 w310]
          tunnel: w302 -> [_ w308]
          tunnel: w301 -> [_ w307]
          frame False {
          }
          frame True {
            # "Update Changed Libraries List."
            n130 = call "ReadHawkeyePathConfig.vi"("error in (no error)"=w310, "Workspace Path"=w311) -> ("error out"=w309:errorcluster, "Hawkeye Path Config Out"=w315:T5)  [unwired: 8 in]
            n131 = Unbundle By Name(w315) -> ("ChangedFilesLogpaths"=w313:map{string, path})
            n132 = Look In Map(map=w313, key="InScopeChangedLVFilesPath") -> (value=w312:path)  [unwired: 1 in, 1 out]
            n133 = call "GenerateChangedFilesList.vi"("GUI Mode? {F)"=w316, "Output File Path"=w312, "error in (no error)"=w309, "Branch 2"=w307, "Branch 1"=w308, "Workspace Path"=w311) -> ("error out"=w318:errorcluster)  [unwired: 5 in]
            n134 = call "GenerateChangedLibrariesList.vi"("GUI Mode? {F)"=w316, "error in (no error)"=w318, "Workspace Path"=w311) -> ("error out"=w317:errorcluster)  [unwired: 8 in]
          }
        }
        n135 = control-ref of="Status Indicator"() -> (w294:refnum<vi>)
        n136 = property class="Str"(reference=w294, error in=w300, "Value"="") -> (error out=w295:errorcluster)  [unwired: 1 out]
        n137 = call "Generate Hawkeye File.vi"("Status Indicator Ref"=w294, "error in (no error)"=w295, "Check Changed Libraries Only?"=w298, "LVLib / LVClass / Folder Path"=w297, "Repo Folder Path"=w296) -> ("error out"=w299:errorcluster)  [unwired: 5 in, 1 out]
      }
      frame "RegenerateHawkeyeList" {
        w319 = ""  # Empty String Constant
        w323 = TRUE  # GUI Mode? {F)
        # "Regenerate Hawkeye List - Get all Lib & Orphan class from from selected repo /workspace update the deps list in HawkeyeList"
        n138 = control-ref of="Status Indicator"() -> (w320:refnum<vi>)
        n139 = property class="Str"(reference=w320, error in=w324, "Value"=w319) -> (error out=w321:errorcluster)  [unwired: 1 out]
        n140 = Unbundle By Name(w328) -> ("Repository Path"=w327:path, "Check Changed Libraries Only?"=w326:bool)
        n141 = control-ref of="Current Status"() -> (w322:refnum<vi>)
        n142 = call "UpdateActualDepsList.vi"("Overall Status Indicator Ref"=w320, "GUI Mode? {F)"=w323, "Current Status Indicator Ref"=w322, "error in (no error)"=w321, "UpdateForChangedLibrariesOnly"=w326, "Workspace Path"=w327) -> ("error out"=w325:errorcluster)  [unwired: 5 in]
      }
      frame "Stop" {
        # "Performs actions when the VI is stopped."
        n143 = for {
          tunnel: string[] ["Exit"] -> [w335] mode=indexing
          shift-right: [w337] -> w332
          shift-left: w333 -> [w338]
          shift-right: [w334] -> _
          shift-left: w331 -> [w336]
          n144 = Enqueue Element(queue=w336, element=w335, error in (no error)=w338) -> (queue out=w334:refnum<queue>, error out=w337:errorcluster)  [unwired: 1 in, 1 out]
        }
      }
      frame "Exit" {
        w341 = TRUE  # Exit?
        # "Finish the execution"
        n145 = Release Queue(queue=w340, error in (no error)=w343) -> (error out=w339:errorcluster)  [unwired: 1 in, 2 out]
      }
      frame "Error" {
        # "In case of any Git API initialization errors, we need to disable the controls."
        # "Show the error dialog and clear out the operations. Update controls status."
        n146 = call <vilib>:"Simple Error Handler.vi"("error in (no error)"=w351) -> ("error out"=w350:errorcluster)  [unwired: 4 in, 4 out]
        n147 = call <vilib>:"Clear Errors.vi"("error in (no error)"=w350) -> ("error out"=w349:errorcluster)  [unwired: 5 in, 1 out]
        n148 = Flush Queue(queue=w348, error in (no error)=w349) -> (queue out=w345:refnum<queue>, error out=w346:errorcluster)  [unwired: 1 out]
        n149 = for {
          tunnel: string[] ["Enable Disable Controls"] -> [w354] mode=indexing
          shift-right: [w356] -> w344
          shift-left: w346 -> [w357]
          shift-right: [w353] -> _
          shift-left: w345 -> [w355]
          n150 = Enqueue Element(queue=w355, element=w354, error in (no error)=w357) -> (queue out=w353:refnum<queue>, error out=w356:errorcluster)  [unwired: 1 in, 1 out]
        }
      }
    }
  }
  n151 = invoke class="VI" method="FP.Close"(error in=w4) -> (error out=w3:errorcluster)  [unwired: 2 in, 2 out]
  n152 = call <vilib>:"Clear Errors.vi"("error in (no error)"=w3) -> ()  [unwired: 5 in, 2 out]
